vi "Finalize.vi"(8 "error in":errorcluster, 11 "Plugin in":refnum<class "Historical Table.lvclass">) -> (0 "error out":errorcluster, 3 "Plugin out":refnum<class "Historical Table.lvclass">)   [LabVIEW 2024, in "Historical Table.lvlib" / "Historical Table.lvclass"]
uses:
  Historical Table.lvclass
  Historical Table.lvclass/Historical Table.ctl
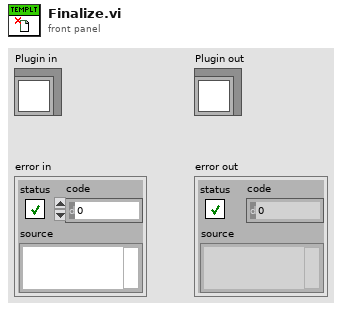
[diagram p1: front panel]
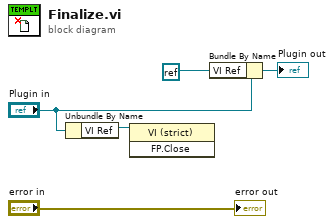
[diagram p0: block diagram]
diagram:
  n1 = Unbundle By Name("Plugin in") -> ("VI Ref"=w4:refnum<vi>)
  n2 = invoke class="VI (strict)" method="FP.Close"(reference=w4) -> ()  [unwired: 2 in, 3 out]
  n3 = Bundle By Name(cluster="Plugin in", "VI Ref"=refnum<k0> refnum) -> (→"Plugin out":refnum<class "Historical Table.lvclass">)
  "error out" <- "error in"
